vi "Main.vi"() -> (0 "error out":errorcluster)   [LabVIEW 2020, in "Program.lvclass"]
uses:
  Program.lvclass
  IFigure_interface/IFigure.lvclass
  Rectangle_class/Rectangle.lvclass
  C:/Projects/DesignPatterns/PrototypePattern/IFigure_interface/IFigure.lvclass
  Circle_class/Circle.lvclass
panel:
  out "appended array":string[](array[string])
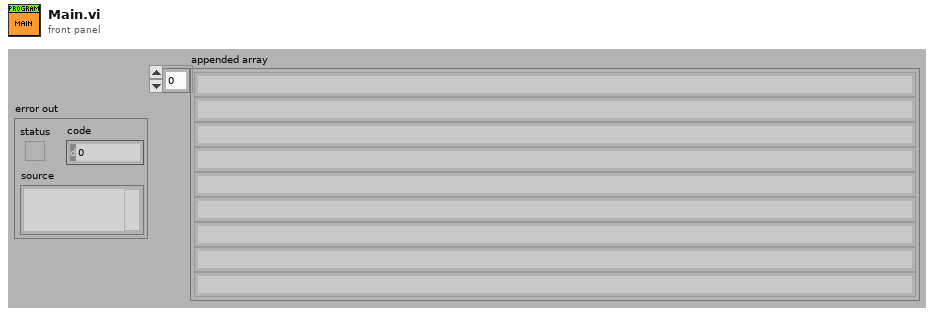
[diagram p1: front panel]
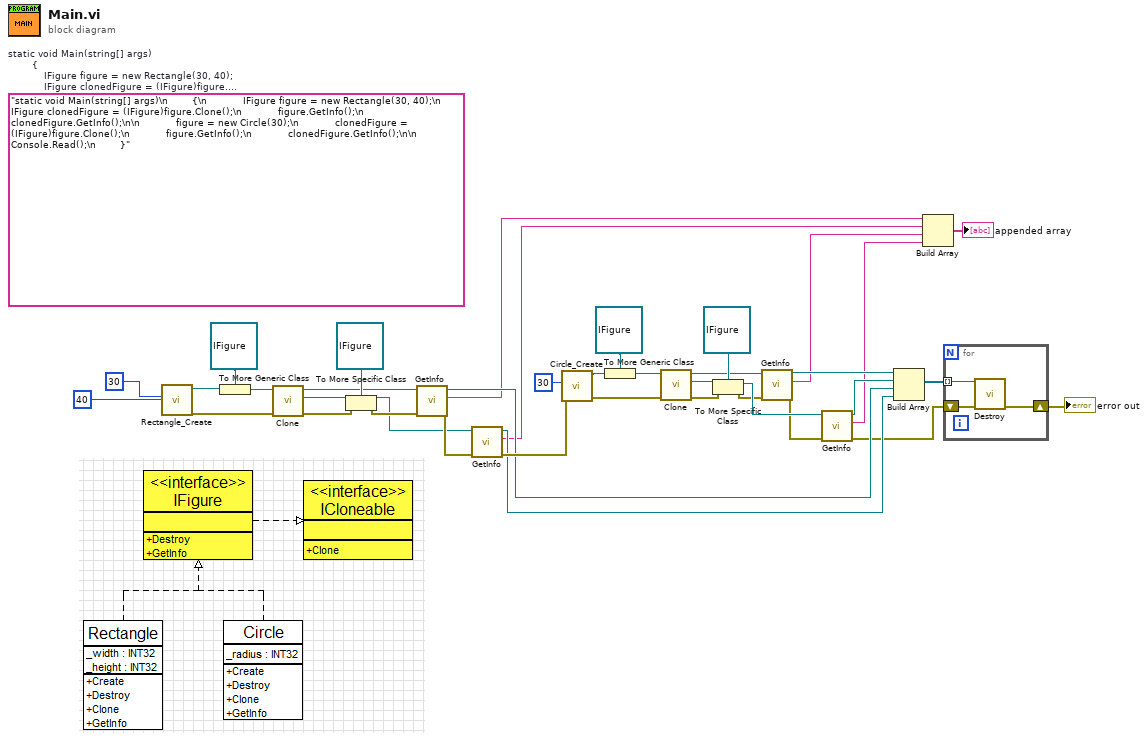
[diagram p0: block diagram]
diagram:
  (unwired) "static void Main(string[] args)\n        {\n            IFigure figure = new Rectangle(30, 40);\n            IFigure clonedFigure = (IFigure)figure.Clone();\n            figure.GetInfo();\n            clonedFigure.GetInfo();\n\n            figure = new Circle(30);\n            clonedFigure = (IFigure)figure.Clone();\n            figure.GetInfo();\n            clonedFigure.GetInfo();\n\n            Console.Read();\n        }"  # static void Main(string[] args)         {             IFigure figure = new Rectangle(30, 40);             IFigure clonedFigure = (IFigure)figure.Clone();             figure.GetInfo();             clonedFigure.GetInfo();              figure = new Circle(30);             clonedFigure = (IFigure)figure.Clone();             figure.GetInfo();             clonedFigure.GetInfo();              Console.Read();         }
  n1 = call "Rectangle_Create.vi"("H"=40, "W"=30) -> ("Error Out"=w27:errorcluster, "reference out"=w36:refnum<class "Rectangle.lvclass">)  [unwired: 8 in]
  n2 = To More Generic Class(target class=refnum<class "IFigure.lvclass"> refnum ("IFigure"), reference=w36) -> (generic class reference=w34:refnum<class "IFigure.lvclass">)
  n3 = call-dynamic "Clone.vi"("Error In"=w27, "object in"=w34) -> ("Error Out"=w28:errorcluster, "Return(LabVIEW Object)"=w33:refnum<class "ICloneable.lvclass">, "object out"=w31:refnum<class "IFigure.lvclass">)  [unwired: 7 in]
  n4 = To More Specific Class(target class=refnum<class "IFigure.lvclass"> refnum ("IFigure"), reference=w33, error in=w28) -> (specific class reference=w26:refnum<class "IFigure.lvclass">, error out=w29:errorcluster)
  n5 = call-dynamic "GetInfo.vi"("Error In"=w29, "object in"=w31) -> ("Error Out"=w30:errorcluster, "Console"=w5:string, "object out"=w10:refnum<class "IFigure.lvclass">)  [unwired: 7 in]
  n6 = call-dynamic "GetInfo.vi"("Error In"=w30, "object in"=w26) -> ("Error Out"=w24:errorcluster, "Console"=w4:string, "object out"=w9:refnum<class "IFigure.lvclass">)  [unwired: 7 in]
  n7 = call "Circle_Create.vi"("Error In"=w24, "R"=30) -> ("Error Out"=w20:errorcluster, "reference out"=w21:refnum<class "Circle.lvclass">)  [unwired: 8 in]
  n8 = To More Generic Class(target class=refnum<class "IFigure.lvclass"> refnum ("IFigure"), reference=w21) -> (generic class reference=w23:refnum<class "IFigure.lvclass">)
  n9 = call-dynamic "Clone.vi"("Error In"=w20, "object in"=w23) -> ("Error Out"=w14:errorcluster, "Return(LabVIEW Object)"=w18:refnum<class "ICloneable.lvclass">, "object out"=w17:refnum<class "IFigure.lvclass">)  [unwired: 7 in]
  n10 = To More Specific Class(target class=refnum<class "IFigure.lvclass"> refnum ("IFigure"), reference=w18, error in=w14) -> (specific class reference=w16:refnum<class "IFigure.lvclass">, error out=w15:errorcluster)
  n11 = call-dynamic "GetInfo.vi"("Error In"=w15, "object in"=w17) -> ("Error Out"=w13:errorcluster, "Console"=w3:string, "object out"=w12:refnum<class "IFigure.lvclass">)  [unwired: 7 in]
  n12 = call-dynamic "GetInfo.vi"("Error In"=w13, "object in"=w16) -> ("Error Out"=w7:errorcluster, "Console"=w2:string, "object out"=w11:refnum<class "IFigure.lvclass">)  [unwired: 7 in]
  n13 = Build Array(w12, w11, w10, w9) -> (w8:refnum<class "IFigure.lvclass">[])
  n14 = Build Array(w5, w4, w3, w2) -> (→"appended array":string[])
  n15 = for {
    tunnel: w8 -> [w41] mode=indexing
    shift-right: [w39] -> w6
    shift-left: w7 -> [w40]
    n16 = call-dynamic "Destroy.vi"("Error In"=w40, "object in"=w41) -> ("Error Out"=w39:errorcluster)  [unwired: 8 in, 1 out]
  }
  "error out" <- w6
